vi "lab4_usrp_cp_ofdm_transceiver.vi"() -> ()   [LabVIEW 2014]
uses:
  <vilib>/addons/Modulation/Digital/General/MT Generate Bits (Galois, PN Order).vi
  <vilib>/Analysis/2dsp.llb/Inverse Real FFT.vi
  <vilib>/Analysis/2dsp.llb/Complex FFT.vi
  <vilib>/Analysis/5stat.llb/RMS (DBL).vi
  <vilib>/addons/Modulation/Digital/Support/Common/Validators/mod_Generate Bits Validate.vi
  <vilib>/addons/Modulation/Analog/support/mod_Set Error Source.vi
  var_stop.vi
  <vilib>/addons/Modulation/Digital/Support/Common/Validators/mod_Generate Filter Coefficients Validate.vi
  <vilib>/addons/Modulation/Digital/General/subVIs/mod_Generate Filter Coefficients.vi
  <vilib>/addons/Modulation/Digital/General/subVIs/mod_Generate Bits PN Sequence.vi
  <vilib>/addons/Modulation/Digital/General/MT Generate QAM System Parameters(M).vi
  <vilib>/addons/Modulation/Digital/General/MT Apply Pulse Shaping Filter (Generic).vi
  <instrlib>/niUSRP/niUSRP Write Tx Data (CDB Cluster).vi
  <vilib>/addons/Modulation/Digital/General/MT Apply Matched Filter (Generic).vi
  <vilib>/addons/Modulation/Digital/General/MT Align to Ideal Symbols (Generic).vi
  <vilib>/addons/Modulation/Digital/General/MT Map QAM Symbols to Bits.vi
  <instrlib>/niUSRP/niUSRP Fetch Rx Data (CDB Cluster).vi
  <vilib>/addons/Modulation/niDMT.lvlib
  <vilib>/Analysis/NI_AALPro.lvlib
panel:
  in  "M-QAM (16)":i32=16
  out "Waveform Graph":dbl[](graph)
  out "OFDM subcarrier (freq)":dbl[](graph)
  out "PAPR":dbl
  out "TX buffer":i32
  out "RX buffer":i32
  out "avg energy":dbl
  in  "TX on":bool=TRUE
  in  "power scale":dbl format="%#_13g"
  out "acc recieved bits":i32
  out "acc error bits":i32
  out "Packet number":u8
  out "Packet bytes":u32
  out "past 20 error bits":i32[](array[numeric])
  in  "min_len":i32=200
  in  "Threshold":dbl=-61.0 format="%#_13g"
  out "Accumulated BER":dbl
  out "found packet":bool
  in  "total bits (128)":i32=1600 caption="bits per packet"
  in  "message carriers":i32=120
  out "RX  constellation map":cdb[](graph)
  in  "pilot carrier":i32=32
  in  "cyclic length":i32=64
  in  "FFT size":i32=256
  in  "filter length (symbols)":i32=8
  in  "filter parameter":dbl=0.35 format="%.2f"
  in  "samples per symbol (16)":i32=4
  in  "pulse shaping filter (none)":T1(ring)=enum."Root Raised Cos"
  in  "stop":bool
  in  "number of samples":i64=20000
  out "coerced carrier frequency":dbl=2400000000.0 format="%#_6p"
  out "coerced IQ rate":dbl=1000000.0 format="%#_6p"
  in  "Clocking and Synchronization:Reference Frequency Source 2":string(combo)="Internal"
  in  "Clocking and Synchronization:Reference Frequency Source":string(combo)="Internal"
  in  "RX gain":dbl format="%#_6f"
  in  "TX gain":dbl format="%#_6f"
  in  "carrier frequency":dbl=2400000000.0 format="%#_6p"
  in  "IQ rate":dbl=1000000.0 format="%#_6p"
  in  "RX device names":refnum<k15>="192.168.10.3"
  in  "TX device names":refnum<k15>="192.168.10.3"
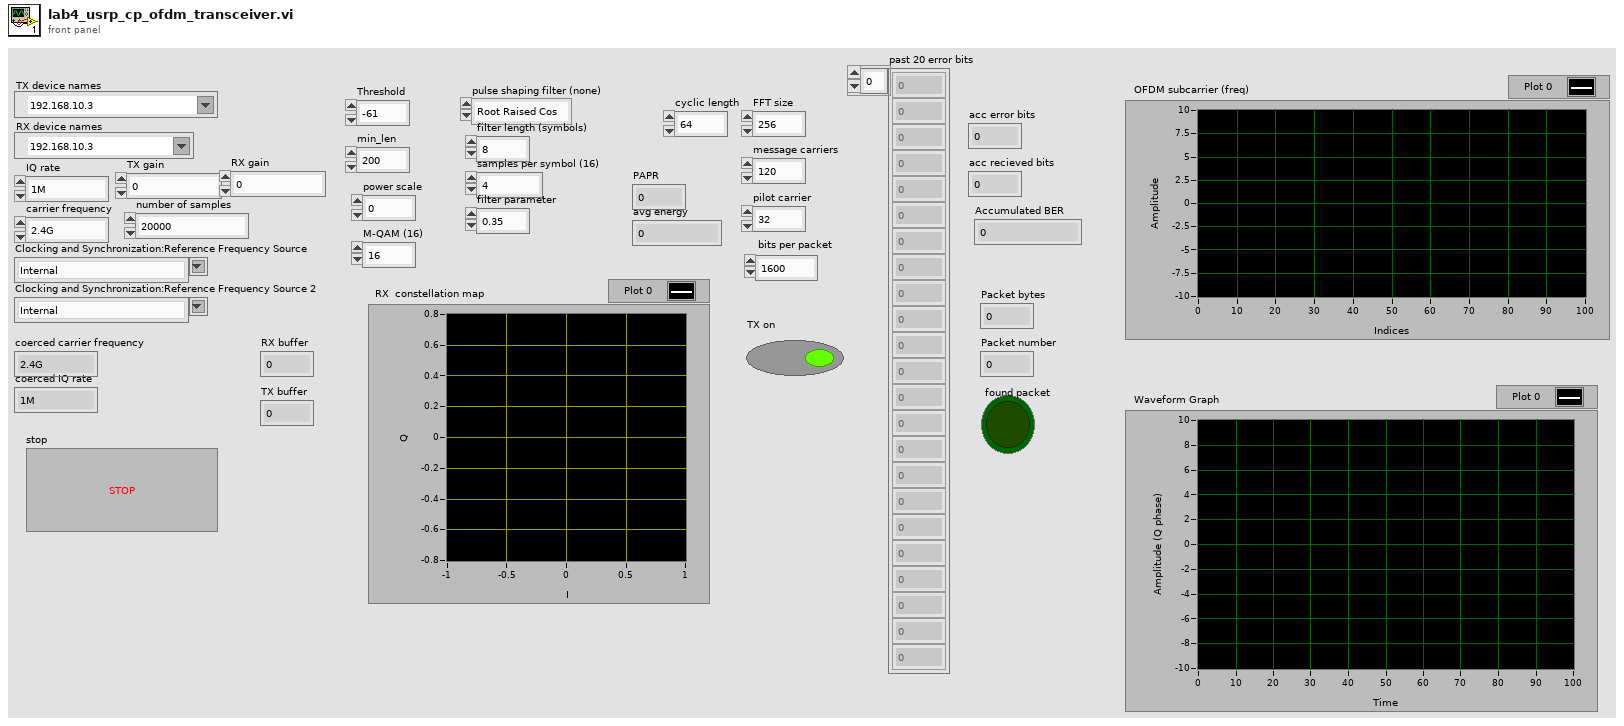
[diagram p1: front panel]
types:
  T1 = enum16{"none", "Raised Cosine", "Root Raised Cos", "Gaussian"}
  T2 = enum16{"FSK", "PSK", "QAM", "MSK", "PAM", "ASK", "CPM"}
  T3 = cluster{"samples per symbol (16)":i32, "symbol map":cdb[]}
  T4 = typedef "niAMT.lvlib/Complex Data Waveform.ctl" = cluster{"t0":dbl, "dt":dbl, "Y":cdb[]}
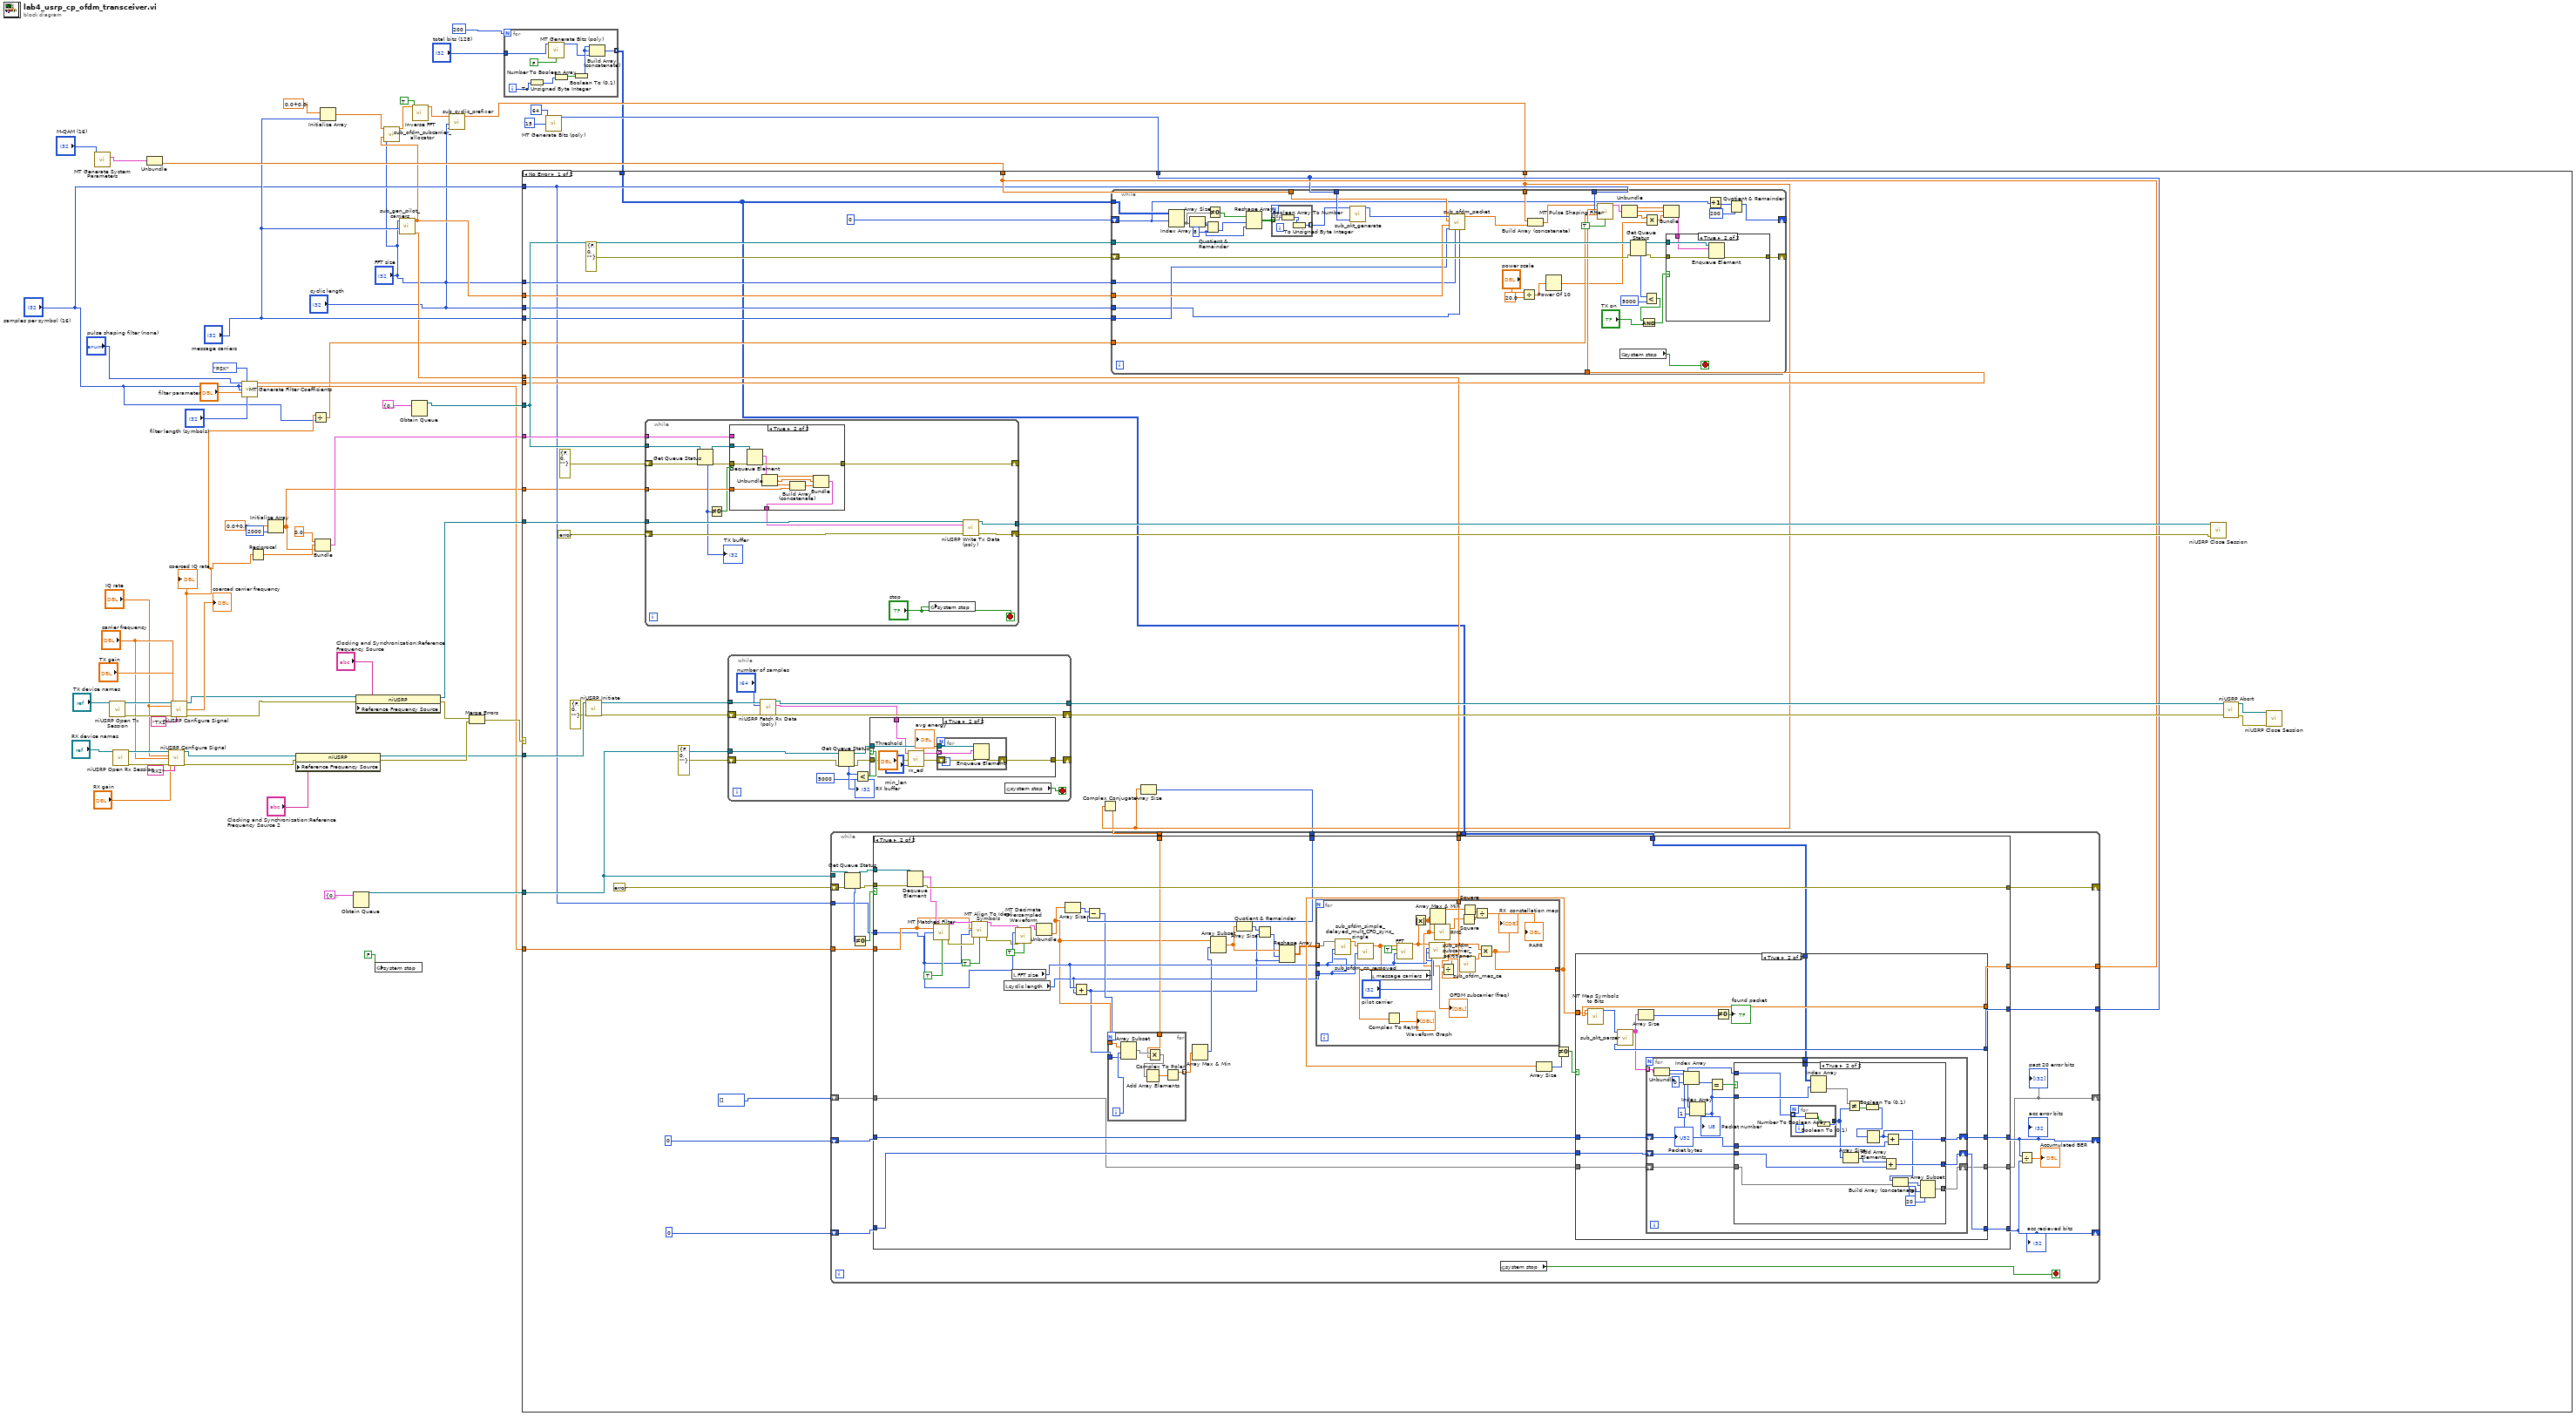
[diagram p0: block diagram]
diagram:
  n1 = call-poly <vilib>:"MT Generate System Parameters.vi"("M-QAM (16)"="M-QAM (16)") -> ("QAM system parameters"=w24:T3)  [unwired: 12 in, 2 out]
  n2 = call <instrlib>:"niUSRP Open Tx Session.vi"("device names"="TX device names") -> ("session handle out"=w64:refnum<k15>, "error out"=w63:errorcluster)  [unwired: 13 in]
  n3 = call <instrlib>:"niUSRP Open Rx Session.vi"("device names"="RX device names") -> ("session handle out"=w60:refnum<k15>, "error out"=w59:errorcluster)  [unwired: 13 in]
  n4 = Unbundle(w24) -> ("symbol map"=w23:cdb[])  [unwired: 1 out]
  n5 = call <instrlib>:"niUSRP Configure Signal.vi"("session handle"=w60, "IQ rate"="IQ rate", "carrier frequency"="carrier frequency", "gain"="RX gain", "error in (no error)"=w59, "active antenna"="RX2") -> ("session handle out"=w51:refnum<k15>, "error out"=w50:errorcluster)  [unwired: 5 in, 3 out]
  n6 = call <instrlib>:"niUSRP Configure Signal.vi"("session handle"=w64, "IQ rate"="IQ rate", "carrier frequency"="carrier frequency", "gain"="TX gain", "error in (no error)"=w63, "active antenna"="TX1") -> ("session handle out"=w26:refnum<k15>, "coerced IQ rate"=w15:dbl, "coerced carrier frequency"=→"coerced carrier frequency":dbl, "error out"=w25:errorcluster)  [unwired: 5 in, 1 out]
  "coerced IQ rate" <- w15
  n7 = call <vilib>:"MT Generate Filter Coefficients.vi"("pulse shaping filter (none)"="pulse shaping filter (none)", "modulation type"=T2."PSK", "pulse shaping samples per symbol (16)"="samples per symbol (16)", "matched samples per symbol (16)"="samples per symbol (16)", "filter parameter"="filter parameter", "filter length (symbols)"="filter length (symbols)") -> ("pulse shaping filter coefficients"=w29:dbl[], "matched filter coefficients"=w28:dbl[])  [unwired: 7 in, 1 out]
  n8 = Reciprocal(x=w15) -> (1/x=w35:dbl)
  n9 = Initialize Array(cdb 0.0+0.0i, 2000 ("dimension size")) -> (w2:cdb[])
  n10 = property class="niUSRP"(reference=w51, error in=w50, "Reference Frequency Source"="Clocking and Synchronization:Reference Frequency Source 2") -> (reference out=w42:refnum<k15>, error out=w46:errorcluster)
  n11 = Divide(x=w15, y="samples per symbol (16)") -> (x/y=w14:dbl)
  n12 = Bundle(0.0, w35, w2) -> (w33:cluster{dbl, dbl, cdb[]})  [unwired: 1 in]
  n13 = Initialize Array(cdb 0.0+0.0i, "message carriers") -> (w18:cdb[])
  n14 = Obtain Queue(element data type=cluster{"t0":dbl, "dt":dbl, "Y":cdb[]} {"t0"=0.0, "dt"=0.0, "Y"=[]} ("data")) -> (queue out=w41:refnum<queue>)  [unwired: 4 in, 2 out]
  n15 = property class="niUSRP"(reference=w26, error in=w25, "Reference Frequency Source"="Clocking and Synchronization:Reference Frequency Source") -> (reference out=w40:refnum<k15>, error out=w47:errorcluster)
  n16 = global write "var_stop.vi" "system stop"(FALSE) -> ()
  n17 = call "sub_gen_pilot_carriers.vi"("message carrier"="message carriers", "FFT size"="FFT size") -> ("RX pilot carriers"=w16:cdb[], "TX pilot carriers"=w12:cdb[])  [unwired: 8 in]
  n18 = call "sub_ofdm_subcarrier_allocator.vi"("fft size"="FFT size", "pilot symbol"=w12, "message symbol"=w18) -> ("OFDM symbol"=w11:cdb[])  [unwired: 8 in]
  n19 = Obtain Queue(element data type=cluster{"t0":dbl, "dt":dbl, "Y":cdb[]} {"t0"=0.0, "dt"=0.0, "Y"=[]} ("data")) -> (queue out=w38:refnum<queue>)  [unwired: 4 in, 2 out]
  n20 = call-poly <vilib>:"Inverse FFT.vi"("shift?"=TRUE, "FFT {X}"=w11) -> ("X"=w9:dbl[])  [unwired: 8 in, 1 out]
  n21 = call "sub_cyclic_prefixer.vi"("FFT size"="FFT size", "CP length"="cyclic length", "time_samples"=w9) -> ("cp ofdm symbol"=w6:cdb[])  [unwired: 8 in]
  n22 = Merge Errors(w47, w46) -> (w45:errorcluster)
  n23 = for {
    N: 200 ("y") -> [_]
    tunnel: "total bits (128)" -> [w72]
    tunnel: [w65] -> w3 mode=indexing
    i -> [w70]
    n24 = To Unsigned Byte Integer(number=w70) -> (unsigned 8bit integer=w69:u8)
    n25 = call-poly <vilib>:"MT Generate Bits (poly).vi"("total bits (128)"=w72, "reset? (T)"=FALSE) -> ("output bit stream"=w66:i8[])  [unwired: 11 in, 2 out]
    n26 = Number To Boolean Array(number=w69) -> (Boolean array=w68:bool[])
    n27 = Boolean To (0,1)(Boolean=w68) -> (0, 1=w67:i16[])
    n28 = Build Array (concatenate)(w67, w67, w66) -> (w65:i16[])
  }
  n29 = call-poly <vilib>:"MT Generate Bits (poly).vi"("total bits (128)"=64, "PN sequence order (9)"=15) -> ("output bit stream"=w20:i8[])  [unwired: 11 in, 2 out]
  n30 = case shown="No Error" w45 {
    tunnel: w42 -> [w109 _]
    tunnel: w41 -> [w104 _]
    tunnel: w40 -> [w99 _]
    tunnel: w38 -> [w96 _]
    tunnel: w33 -> [w97 _]
    tunnel: w29 -> [w94 _]
    tunnel: w28 -> [w93 _]
    tunnel: "message carriers" -> [w90 _]
    tunnel: "FFT size" -> [w89 _]
    tunnel: w23 -> [w88 _]
    tunnel: w20 -> [w87 _]
    tunnel: w16 -> [w86 _]
    tunnel: w14 -> [w85 _]
    tunnel: "samples per symbol (16)" -> [w82 _]
    tunnel: w12 -> [w84 _]
    tunnel: "cyclic length" -> [w83 _]
    tunnel: w6 -> [w76 _]
    tunnel: w3 -> [w80 _]
    tunnel: w2 -> [w77 _]
    frame No Error {
      n31 = call <instrlib>:"niUSRP Initiate.vi"("session handle"=w109, "error in (no error)"=errorcluster {"status"=FALSE, "code"=0, "source"=""}) -> ("session handle out"=w111:refnum<k15>, "error out"=w110:errorcluster)  [unwired: 12 in]
      n32 = while {
        tunnel: [w362] -> w102
        shift-right: [w361] -> w101
        shift-left: errorcluster {"status"=FALSE, "code"=0, "source"=""} ("error out") -> [w359]
        tunnel: w99 -> [w360]
        tunnel: w96 -> [w358]
        shift-right: [w352] -> _
        shift-left: errorcluster {"status"=FALSE, "code"=0, "source"=""} ("error out") -> [w357]
        tunnel: w97 -> [w351]
        tunnel: w77 -> [w350]
        stop <- "stop" stop-if-true
        n33 = Get Queue Status(queue=w358, error in (no error)=w357) -> (queue out=w354:refnum<queue>, error out=w355:errorcluster, # elements in queue=w356:i32)  [unwired: 1 in, 5 out]
        "TX buffer" <- w356
        n34 = Not Equal To 0?(x=w356) -> (x != 0?=w349:bool)
        n35 = case shown="True" w349 {
          tunnel: w355 -> [w365 w374]
          tunnel: w354 -> [_ w375]
          tunnel: [w364 w366] -> w353
          tunnel: [w365 w373] -> w352
          tunnel: w351 -> [w364 _]
          tunnel: w350 -> [_ w370]
          frame False {
          }
          frame True {
            n36 = Dequeue Element(queue=w375, error in (no error)=w374) -> (element=w372:cluster{"t0":dbl, "dt":dbl, "Y":cdb[]}, error out=w373:errorcluster)  [unwired: 1 in, 2 out]
            n37 = Unbundle(w372) -> ("t0"=w367:dbl, "dt"=w368:dbl, "Y"=w371:cdb[])
            n38 = Build Array (concatenate)(w371, w370) -> (w369:cdb[])
            n39 = Bundle("t0"=w367, "dt"=w368, w369) -> (w366:cluster{"t0":dbl, "dt":dbl, cdb[]})  [unwired: 1 in]
          }
        }
        n40 = global write "var_stop.vi" "system stop"("stop") -> ()
        n41 = call-poly <instrlib>:"niUSRP Write Tx Data (poly).vi"("session handle"=w360, "data"=w353, "error in (no error)"=w359) -> ("session handle out"=w362:refnum<k15>, "error out"=w361:errorcluster)  [unwired: 11 in]
      }
      n42 = while {
        tunnel: w111 -> [w335]
        shift-right: [w328] -> w106
        shift-left: w110 -> [w334]
        tunnel: [w329] -> w107
        tunnel: w104 -> [w325]
        shift-right: [w323] -> _
        shift-left: errorcluster {"status"=FALSE, "code"=0, "source"=""} ("error out") -> [w322]
        stop <- w321 stop-if-true
        n43 = call-poly <instrlib>:"niUSRP Fetch Rx Data (poly).vi"("session handle"=w335, "number of samples"="number of samples", "error in (no error)"=w334) -> ("session handle out"=w329:refnum<k15>, "data"=w327:cluster{"t0":dbl, "dt":dbl, "Y":cdb[]}, "error out"=w328:errorcluster)  [unwired: 9 in, 1 out]
        n44 = Get Queue Status(queue=w325, error in (no error)=w322) -> (queue out=w326:refnum<queue>, error out=w324:errorcluster, # elements in queue=w332:i32)  [unwired: 1 in, 5 out]
        "RX buffer" <- w332
        n45 = Less?(x=w332, y=5000) -> (x < y?=w330:bool)
        n46 = case shown="True" w330 {
          tunnel: w327 -> [_ w341]
          tunnel: w326 -> [_ w342]
          tunnel: w324 -> [w336 w344]
          tunnel: [w336 w343] -> w323
          frame False {
          }
          frame True {
            n47 = call "rx_ed.vi"("min_len"="min_len", "Threshold"="Threshold", "Wavefrom"=w341) -> ("avg energy"=→"avg energy":dbl, "extract wav"=w338:cluster{"t0":dbl, "dt":dbl, cdb[]}[])  [unwired: 7 in]
            n48 = for {
              tunnel: w342 -> [w346]
              shift-right: [w347] -> w343
              shift-left: w344 -> [w348]
              tunnel: w338 -> [w345] mode=indexing
              n49 = Enqueue Element(queue=w346, element=w345, error in (no error)=w348) -> (error out=w347:errorcluster)  [unwired: 1 in, 2 out]
            }
          }
        }
        n50 = global read "var_stop.vi" "system stop"() -> (w321:bool)
      }
      n51 = Complex Conjugate(1:w76) -> (0:w74:cdb[])
      n52 = while {
        tunnel: w96 -> [w151]
        shift-right: [w153] -> _
        shift-left: errorcluster {"status"=FALSE, "code"=0, "source"=""} ("error out") -> [w152]
        tunnel: w84 -> [w143]
        tunnel: w94 -> [w150]
        tunnel: w82 -> [w149]
        tunnel: w85 -> [w148]
        tunnel: w90 -> [w142]
        tunnel: w89 -> [w141]
        tunnel: w88 -> [w144]
        tunnel: w87 -> [w146]
        tunnel: w83 -> [w140]
        tunnel: w76 -> [w139]
        tunnel: w80 -> [w136]
        shift-right: [w132] -> _
        shift-left: 0 -> [w135]
        stop <- w158 stop-if-true
        w129 = 8 ("y")
        n53 = Index Array(array=w136, index (row)=w135) -> (element=w128:i16[])  [unwired: 1 in]
        n54 = Array Size(array=w128) -> (size(s)=w131:i32)
        n55 = Quotient & Remainder(x=w131, y=w129) -> (floor(x/y)=w130:i32)  [unwired: 1 out]
        n56 = Not Equal To 0?(x=w128) -> (x != 0?=w127:bool[])
        n57 = Reshape Array(w127, w130, w129) -> (w126:bool[][])
        n58 = for {
          tunnel: w126 -> [w161] mode=indexing
          tunnel: [w159] -> w125 mode=indexing
          n59 = Boolean Array To Number(Boolean array=w161) -> (number=w160:u32)
          n60 = To Unsigned Byte Integer(number=w160) -> (unsigned 8bit integer=w159:u8)
        }
        n61 = call "sub_pkt_generate.vi"("accesscode (bit)"=w146, "byte stream"=w125) -> ("bit pkt"=w145:i16[])  [unwired: 9 in]
        n62 = call "sub_ofdm_packet.vi"("CP length"=w140, "FFT size"=w141, "message carriers"=w142, "pilot symbol"=w143, "symbol map"=w144, "packet"=w145) -> ("ofdm packet"=w138:cdb[])  [unwired: 5 in]
        n63 = Divide(x="power scale", y=20.0) -> (x/y=w122:dbl)
        n64 = Build Array (concatenate)(w139, w138) -> (w137:cdb[])
        n65 = Power Of 10(x=w122) -> (10^x=w119:dbl)
        n66 = call-poly <vilib>:"MT Pulse Shaping Filter.vi"("symbols"=w137, "pulse shaping filter coefficients"=w150, "samples per symbol (16)"=w149, "symbol rate (Hz)"=w148, "reset? (T)"=TRUE) -> ("output complex waveform"=w121:T4)  [unwired: 9 in, 1 out]
        n67 = global read "var_stop.vi" "system stop"() -> (w158:bool)
        n68 = Unbundle(w121) -> ("t0"=w116:dbl, "dt"=w117:dbl, "Y"=w120:cdb[])
        n69 = Get Queue Status(queue=w151, error in (no error)=w152) -> (queue out=w155:refnum<queue>, error out=w154:errorcluster, # elements in queue=w157:i32)  [unwired: 1 in, 5 out]
        n70 = Less?(x=w157, y=5000) -> (x < y?=w114:bool)
        n71 = And(x=w114, y="TX on") -> (x .and. y?=w112:bool)
        n72 = Multiply(x=w120, y=w119) -> (x*y=w118:cdb[])
        n73 = Bundle("t0"=w116, "dt"=w117, w118) -> (w115:cluster{"t0":dbl, "dt":dbl, cdb[]})  [unwired: 1 in]
        n74 = case shown="True" w112 {
          tunnel: w155 -> [_ w166]
          tunnel: w154 -> [w162 w165]
          tunnel: [w162 w164] -> w153
          tunnel: w115 -> [_ w163]
          frame False {
          }
          frame True {
            n75 = Enqueue Element(queue=w166, element=w163, error in (no error)=w165) -> (error out=w164:errorcluster)  [unwired: 1 in, 2 out]
          }
        }
        n76 = Increment(x=w135) -> (x+1=w134:i32)
        n77 = Quotient & Remainder(x=w134, y=200) -> (x-y*floor(x/y)=w132:i32)  [unwired: 1 out]
      }
      n78 = Array Size(array=w76) -> (size(s)=w75:i32)
      n79 = while {
        tunnel: w104 -> [w184]
        shift-right: [w182] -> _
        shift-left: errorcluster {"status"=FALSE, "code"=0, "source"=""} ("error out") -> [w183]
        tunnel: w93 -> [w181]
        tunnel: w82 -> [w180]
        tunnel: w86 -> [w179]
        tunnel: w88 -> [w178]
        tunnel: w87 -> [w177]
        tunnel: w80 -> [w176]
        shift-right: [w172] -> _
        shift-left: 0 -> [w174]
        shift-right: [w173] -> _
        shift-left: 0 -> [w175]
        tunnel: w75 -> [w170]
        tunnel: w74 -> [w169]
        shift-right: [w167] -> _
        shift-left: i32[] [] -> [w168]
        stop <- w189 stop-if-true
        n80 = Get Queue Status(queue=w184, error in (no error)=w183) -> (queue out=w185:refnum<queue>, error out=w186:errorcluster, # elements in queue=w188:i32)  [unwired: 1 in, 5 out]
        n81 = Not Equal To 0?(x=w188) -> (x != 0?=w187:bool)
        n82 = case shown="True" w187 {
          tunnel: w186 -> [w193 w234]
          tunnel: w185 -> [_ w233]
          tunnel: [w193 w232] -> w182
          tunnel: w181 -> [_ w224]
          tunnel: w180 -> [_ w223]
          tunnel: w179 -> [_ w227]
          tunnel: w178 -> [_ w219]
          tunnel: w177 -> [_ w218]
          tunnel: w176 -> [_ w217]
          tunnel: w175 -> [w192 w216]
          tunnel: w174 -> [w191 w215]
          tunnel: [w192 w214] -> w173
          tunnel: [w191 w213] -> w172
          tunnel: w170 -> [_ w208]
          tunnel: w169 -> [_ w204]
          tunnel: w168 -> [w190 w195]
          tunnel: [w190 w194] -> w167
          frame False {
          }
          frame True {
            n83 = Dequeue Element(queue=w233, error in (no error)=w234) -> (element=w231:cluster{"t0":dbl, "dt":dbl, "Y":cdb[]}, error out=w232:errorcluster)  [unwired: 1 in, 2 out]
            n84 = call-poly <vilib>:"MT Matched Filter.vi"("input complex waveform"=w231, "matched filter coefficients"=w224, "samples per symbol (16)"=w223, "reset? (T)"=TRUE) -> ("output complex waveform"=w226:T4, "error out"=w225:errorcluster)  [unwired: 10 in]
            n85 = call-poly <vilib>:"MT Align To Ideal Symbols.vi"("input complex waveform"=w226, "matched filter coefficients"=w224, "samples per symbol (16)"=w223, "error in (no error)"=w225, "reset? (T)"=TRUE) -> ("output complex waveform"=w221:T4, "error out"=w220:errorcluster)  [unwired: 8 in, 1 out]
            n86 = local read "cyclic length"() -> (w205:i32)
            n87 = local read "FFT size"() -> (w206:i32)
            n88 = call <vilib>:"MT Decimate Oversampled Waveform.vi"("input complex waveform"=w221, "decimation factor"=w223, "error in (no error)"=w220, "reset? (T)"=TRUE) -> ("output complex waveform"=w229:T4)  [unwired: 10 in, 1 out]
            n89 = Unbundle(w229) -> ("Y"=w202:cdb[])  [unwired: 2 out]
            n90 = Array Size(array=w202) -> (size(s)=w209:i32)
            n91 = Add(x=w206, y=w205) -> (x+y=w197:i32)
            n92 = Subtract(x=w209, y=w208) -> (x-y=w207:i32)
            n93 = for {
              N: w207 -> [_]
              tunnel: w202 -> [w242]
              tunnel: w197 -> [w240]
              tunnel: w204 -> [w238]
              tunnel: [w235] -> w203 mode=indexing
              i -> [w241]
              n94 = Array Subset(array=w242, index=w241, length=w240) -> (w239:cdb[])
              n95 = Multiply(x=w239, y=w238) -> (x*y=w237:cdb[])
              n96 = Add Array Elements(numeric array=w237) -> (sum=w236:cdb)
              n97 = Complex To Polar(r * e^(i*theta)=w236) -> (r=w235:dbl)  [unwired: 1 out]
            }
            n98 = Array Max & Min(array=w203) -> (max index (indices)=w201:i32)  [unwired: 3 out]
            n99 = Array Subset(array=w202, index=w201) -> (w199:cdb[])  [unwired: 1 in]
            n100 = Array Size(array=w199) -> (size(s)=w200:i32)
            n101 = Quotient & Remainder(x=w200, y=w197) -> (floor(x/y)=w198:i32)  [unwired: 1 out]
            n102 = Reshape Array(w199, w198, w197) -> (w196:cdb[][])
            n103 = for {
              tunnel: w196 -> [w311] mode=indexing
              tunnel: w205 -> [w308]
              tunnel: w206 -> [w309]
              tunnel: [w317] -> w212 mode=concatenating
              tunnel: w227 -> [w314]
              n104 = call "sub_ofdm_simple_delayed_mult_CFO_sync_single.vi"("CP length"=w308, "FFT size"=w309, "time samples"=w311) -> ("sync ofdm symbol"=w310:cdb[])  [unwired: 8 in]
              n105 = call "sub_ofdm_cp_removed.vi"("CP length"=w308, "time ofdm symbol"=w310) -> ("cp removed ofdm symbol"=w300:cdb[])  [unwired: 9 in]
              n106 = local read "message carriers"() -> (w316:i32)
              n107 = Complex To Re/Im(x + iy=w300) -> (y=→"Waveform Graph":dbl[])  [unwired: 1 out]
              n108 = call-poly <vilib>:"FFT.vi"("FFT size"=w309, "shift?"=TRUE, "X"=w300) -> ("FFT {X}"=w307:cdb[])  [unwired: 7 in, 1 out]
              n109 = Absolute Value(x=w307) -> (abs(x)=w301:dbl[])
              "OFDM subcarrier (freq)" <- w301
              n110 = call "sub_ofdm_subcarrier_partitioner.vi"("pilot carrier"="pilot carrier", "message carrier"=w316, "FFT size"=w309, "received symbol"=w307) -> ("pilot subcarriers"=w313:cdb[], "message subcarriers"=w315:cdb[])  [unwired: 6 in]
              n111 = Array Max & Min(array=w301) -> (max value=w306:dbl)  [unwired: 3 out]
              n112 = call-poly <vilib>:"RMS.vi"("X"=w301) -> ("rms value"=w305:dbl)  [unwired: 1 out]
              n113 = Divide(x=w314, y=w313) -> (x/y=w312:cdb[])
              n114 = call "sub_ofdm_mes_ce.vi"("ZF channel estimates"=w312) -> ("interpolated mes carrier CE"=w318:cdb[])  [unwired: 10 in]
              n115 = Square(x=w305) -> (x^2=w303:dbl)
              n116 = Square(x=w306) -> (x^2=w304:dbl)
              n117 = Divide(x=w304, y=w303) -> (x/y=→"PAPR":dbl)
              n118 = Multiply(x=w315, y=w318) -> (x*y=w317:cdb[])
              "RX  constellation map" <- w317
            }
            n119 = Array Size(array=w212) -> (size(s)=w211:i32)
            n120 = Not Equal To 0?(x=w211) -> (x != 0?=w210:bool)
            n121 = case shown="True" w210 {
              tunnel: w219 -> [_ w259]
              tunnel: w218 -> [_ w257]
              tunnel: w217 -> [_ w253]
              tunnel: w216 -> [w245 w252]
              tunnel: w215 -> [w244 w251]
              tunnel: [w245 w250] -> w214
              tunnel: [w244 w249] -> w213
              tunnel: w212 -> [_ w248]
              tunnel: w195 -> [w243 w247]
              tunnel: [w243 w246] -> w194
              frame False {
              }
              frame True {
                n122 = call-poly <vilib>:"MT Map Symbols to Bits.vi"("symbols"=w248, "symbol map"=w259) -> ("output bit stream"=w258:i8[])  [unwired: 12 in, 1 out]
                n123 = call "sub_pkt_parser.vi"("accesscode (bit)"=w257, "bitstream"=w258) -> ("parsed packet"=w254:cluster{"t":u32, "byte_array":u8[]}[])  [unwired: 9 in]
                n124 = Array Size(array=w254) -> (size(s)=w256:i32)
                n125 = for {
                  tunnel: w254 -> [w274] mode=indexing
                  tunnel: w253 -> [w268]
                  shift-right: [w265] -> w250
                  shift-left: w252 -> [w266]
                  shift-right: [w263] -> w249
                  shift-left: w251 -> [w264]
                  shift-right: [w261] -> w246
                  shift-left: w247 -> [w262]
                  n126 = Unbundle(w274) -> ("t"=→"Packet bytes":u32, "byte_array"=w269:u8[])
                  n127 = Index Array(array=w269, index=0) -> (element=w271:u8)
                  n128 = Index Array(array=w269, index=1) -> (element=w267:u8)
                  "Packet number" <- w267
                  n129 = Equal?(x=w271, y=w267) -> (x = y?=w270:bool)
                  n130 = case shown="True" w270 {
                    tunnel: w269 -> [_ w278]
                    tunnel: w268 -> [_ w295]
                    tunnel: w267 -> [_ w294]
                    tunnel: w266 -> [w277 w290]
                    tunnel: [w277 w289] -> w265
                    tunnel: w264 -> [w276 w286]
                    tunnel: [w276 w285] -> w263
                    tunnel: w262 -> [w275 w284]
                    tunnel: [w275 w279] -> w261
                    frame False {
                    }
                    frame True {
                      n131 = for {
                        tunnel: w278 -> [w298] mode=indexing
                        tunnel: [w296] -> w288 mode=concatenating
                        n132 = Number To Boolean Array(number=w298) -> (Boolean array=w297:bool[])
                        n133 = Boolean To (0,1)(Boolean=w297) -> (0, 1=w296:i16[])
                      }
                      n134 = Index Array(array=w295, index (row)=w294) -> (element=w293:i16[])  [unwired: 1 in]
                      n135 = Array Size(array=w288) -> (size(s)=w287:i32)
                      n136 = Not Equal?(x=w293, y=w288) -> (x != y?=w292:bool[])
                      n137 = Boolean To (0,1)(Boolean=w292) -> (0, 1=w291:i16[])
                      n138 = Add Array Elements(numeric array=w291) -> (sum=w283:i16)
                      n139 = Add(x=w287, y=w286) -> (x+y=w285:i32)
                      n140 = Add(x=w283, y=w290) -> (x+y=w289:i32)
                      n141 = Build Array (concatenate)(w283, w284) -> (w282:i32[])
                      n142 = Array Subset(array=w282, index=0, length=20) -> (w279:i32[])
                    }
                  }
                }
                n143 = Not Equal To 0?(x=w256) -> (x != 0?=→"found packet":bool)
              }
            }
          }
        }
        "past 20 error bits" <- w167
        "acc error bits" <- w173
        "acc recieved bits" <- w172
        n144 = global read "var_stop.vi" "system stop"() -> (w189:bool)
        n145 = Divide(x=w173, y=w172) -> (x/y=→"Accumulated BER":dbl)
      }
      n146 = call <instrlib>:"niUSRP Close Session.vi"("session handle"=w102, "error in (no error)"=w101) -> ()  [unwired: 13 in, 1 out]
      n147 = call <instrlib>:"niUSRP Abort.vi"("session handle"=w107, "error in (no error)"=w106) -> ("session handle out"=w92:refnum<k15>, "error out"=w91:errorcluster)  [unwired: 12 in]
      n148 = call <instrlib>:"niUSRP Close Session.vi"("session handle"=w92, "error in (no error)"=w91) -> ()  [unwired: 13 in, 1 out]
    }
    frame Error {
    }
  }
